vi "get ids.vi"(8 "error in (no error)":errorcluster, 9 "id_size":u16, 10 "nb":u16, 11 "identifier":string) -> (0 "error out":errorcluster, 1 "id_size out":u16, 2 "nb out":u16, 3 "identifier out":string, 5 "function return":bool)   [LabVIEW 2015, in "XGL_DPP.lvlib"]
doc: "EXTERN DECLSPEC bool CALL_CONV get_ids(char* identifier, unsigned short int& nb, unsigned short int& id_size);"
uses:
  XGL_DPP.lvlib
  XGL_DPP.dll
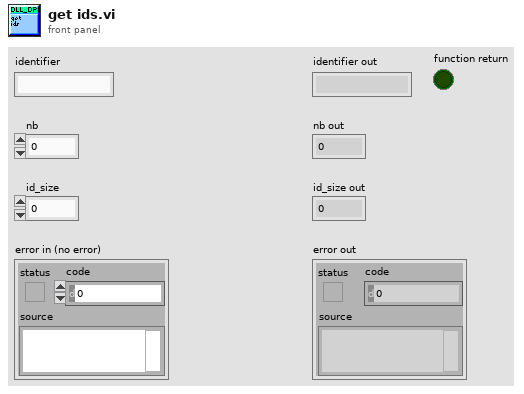
[diagram p1: front panel]
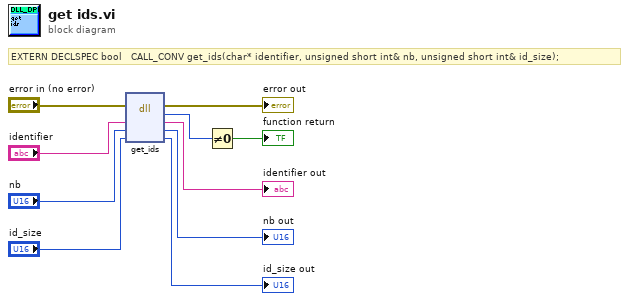
[diagram p0: block diagram]
diagram:
  # "EXTERN DECLSPEC bool   CALL_CONV get_ids(char* identifier, unsigned short int& nb, unsigned short int& id_size);"
  n1 = dll-call lib="D:/Users/XRF/Desktop/Dante_acquire4/libs/Dante/XGL_DPP.*" fn="get_ids"(error in="error in (no error)", "identifier"="identifier", "nb"="nb", "id_size"="id_size") -> (error out=→"error out":errorcluster, "return type"=w9:u8, "identifier"=→"identifier out":string, "nb"=→"nb out":u16, "id_size"=→"id_size out":u16)  [unwired: 2 in, 1 out]
  n2 = Not Equal To 0?(x=w9) -> (x != 0?=→"function return":bool)
